vi "Apply Plot Property.vi"(6 "Plot ID":i32, 8 "error in (no error)":errorcluster, 9 "Plot Property":T1, 11 "Polar Area Ref In":refnum<vi>) -> (0 "error out":errorcluster, 3 "Polar Area Ref Out":refnum<vi>)   [LabVIEW 2017, in "2D Plot.lvclass"]
uses:
  <vilib>/Math Plots/2D Math Plots/2D Plot/2D Plot/2D Plot.lvclass
  <vilib>/Math Plots/2D Math Plots/2D Plot/2D Plot/Typedef/Plot Property.ctl
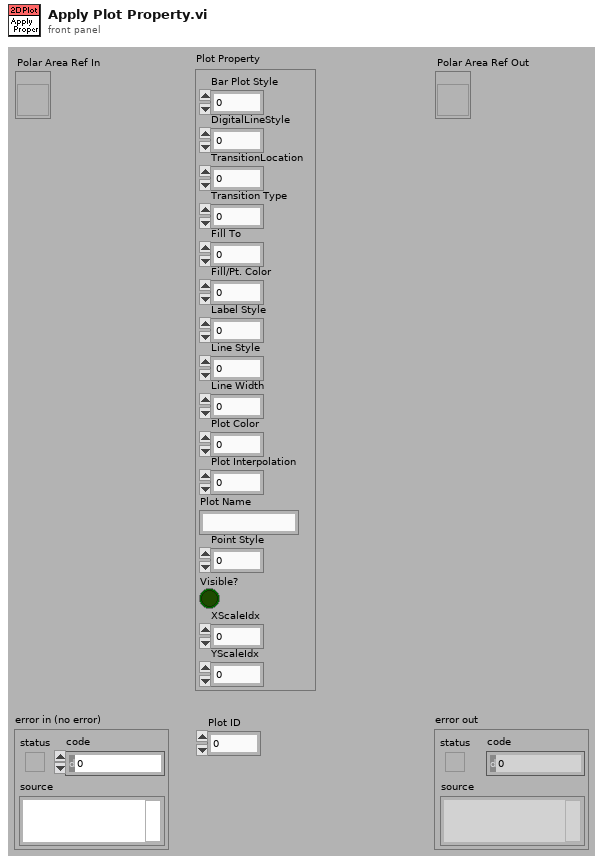
[diagram p1: front panel]
types:
  T1 = typedef "2D Plot.lvclass/Plot Property.ctl" = cluster{"Bar Plot Style":u8, "DigitalLineStyle":u8, "TransitionLocation":u8, "Transition Type":u8, "Fill To":i16, "Fill/Pt. Color":u32, "Label Style":u8, "Line Style":u8, "Line Width":u8, "Plot Color":u32, "Plot Interpolation":u8, "Plot Name":string, "Point Style":u8, "Visible?":bool, "XScaleIdx":u32, "YScaleIdx":u32}
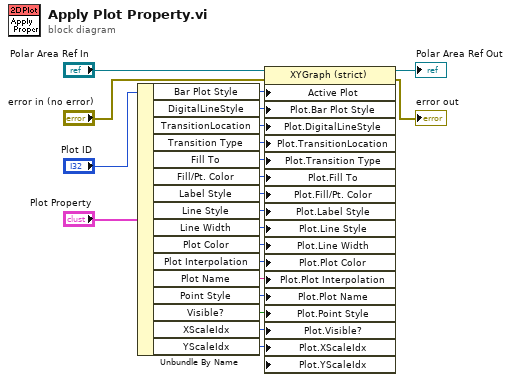
[diagram p0: block diagram]
diagram:
  n1 = Unbundle By Name("Plot Property") -> ("Bar Plot Style"=w19:u8, "DigitalLineStyle"=w18:u8, "TransitionLocation"=w17:u8, "Transition Type"=w16:u8, "Fill To"=w15:i16, "Fill/Pt. Color"=w6:u32, "Label Style"=w7:u8, "Line Style"=w5:u8, "Line Width"=w8:u8, "Plot Color"=w9:u32, "Plot Interpolation"=w14:u8, "Plot Name"=w10:string, "Point Style"=w4:u8, "Visible?"=w3:bool, "XScaleIdx"=w13:u32, "YScaleIdx"=w11:u32)
  n2 = property class="XYGraph (strict)"(reference="Polar Area Ref In", error in="error in (no error)", "Active Plot"="Plot ID", "Plot.Bar Plot Style"=w19, "Plot.DigitalLineStyle"=w18, "Plot.TransitionLocation"=w17, "Plot.Transition Type"=w16, "Plot.Fill To"=w15, "Plot.Fill/Pt. Color"=w6, "Plot.Label Style"=w7, "Plot.Line Style"=w5, "Plot.Line Width"=w8, "Plot.Plot Color"=w9, "Plot.Plot Interpolation"=w14, "Plot.Plot Name"=w10, "Plot.Point Style"=w4, "Plot.Visible?"=w3, "Plot.XScaleIdx"=w13, "Plot.YScaleIdx"=w11) -> (reference out=→"Polar Area Ref Out":refnum<vi>, error out=→"error out":errorcluster)
